vi "Prop Set.vi"(9 "Data Name":string="Value", 10 "Control":refnum<vi>, 11 "Prop":refnum<vi>) -> (3 "Prop out":refnum<vi>)   [LabVIEW 2015]
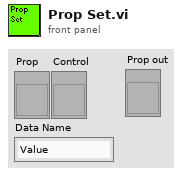
[diagram p1: front panel]
types:
  T1 = typedef "ASPM_ArrayOfUniqueIDStringDatanameShortnameLongname.ctl" = T2[]
  T2 = typedef "ASPM_UniqueIDStringDatanameShortnameLongname.ctl" = cluster{"Unique ID string":string, "Data name":string, "Short name (localized)":string, "Long name (localized)":string}
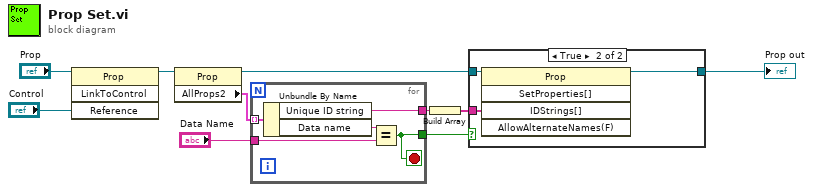
[diagram p0: block diagram]
diagram:
  n1 = invoke class="Prop" method="LinkToControl"(reference="Prop", "Reference"="Control") -> (reference out=w4:refnum<vi>)  [unwired: 2 in, 3 out]
  n2 = property class="Prop"(reference=w4) -> (reference out=w10:refnum<vi>, "AllProps2"=w5:T1)  [unwired: 1 in, 1 out]
  n3 = for {
    tunnel: w5 -> [w15] mode=indexing
    tunnel: "Data Name" -> [w13]
    tunnel: [w12] -> w7
    tunnel: [w11] -> w8
    stop <- w12 stop-if-true
    n4 = Unbundle By Name(w15) -> ("Unique ID string"=w11:string, "Data name"=w14:string)
    n5 = Equal?(x=w14, y=w13) -> (x = y?=w12:bool)
  }
  n6 = Build Array(w8) -> (w9:string[])
  n7 = case shown="True" w7 {
    tunnel: w10 -> [w16 w19]
    tunnel: w9 -> [_ w18]
    tunnel: [w16 w17] -> w1
    frame False {
    }
    frame True {
      n8 = invoke class="Prop" method="SetProperties[]"(reference=w19, "IDStrings[]"=w18) -> (reference out=w17:refnum<vi>)  [unwired: 3 in, 4 out]
    }
  }
  "Prop out" <- w1
